vi "Number of Plots Per Tab - Maximum--Const.vi"() -> (3 "Maximum Plots Per Tab":i32)   [LabVIEW 2017, in "DTacq Plot Display Library.lvlib"]
doc: "The maximum number of plots allowed on a single tab"
uses:
  DTacq Plot Display Library.lvlib
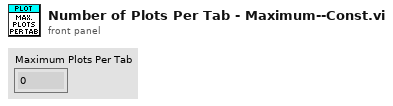
[diagram p1: front panel]
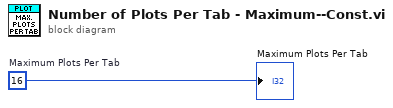
[diagram p0: block diagram]
diagram:
  w1 = 16  # Maximum Plots Per Tab
  "Maximum Plots Per Tab" <- w1
